vi "Flowmeter.vi"() -> ()   [LabVIEW 2018]
panel:
  in  "Doppler Flow Meter Graphs":u16(ring) items=["Ultrasound Speed", "Theta", "Frequency"]
  in  "Speed of Sound in Fluid (m/s)":dbl(knob) scale=0.0..1000.0
  out "XY Graph":cluster{"Y":dbl[], "Y":dbl[]}[](graph)
  in  "Switch 2":bool
  out "?":bool
  out "Velocity":dbl(knob) scale=0.0..5000.0
  in  "Ultrasonic Mode Switch":bool
  in  "?":bool
  in  "Thickness of pipe (mm)":dbl(slide) scale=0.0..200.0
  in  "Magnetic Field (T)":dbl(knob) scale=0.0..1000.0
  in  "Induced EMF (V)":dbl(knob) scale=0.0..10.0
  in  "Angle":dbl(knob) scale=90.0..30.0
  in  "Frequency 1 (KHz)":dbl(knob) scale=0.0..1000.0
  in  "Frequency 2 (KHz)":dbl(knob) scale=0.0..1000.0
  in  "milliseconds to wait":dbl
  in  "?":bool
  # "Variation wrt Difference\n      in Frequency"
  # "Variation wrt Angle"
  # "Electromagnetic"
  # "Ultrasonic"
  # "Doppler Flow Meter"
  # "Transit Time"
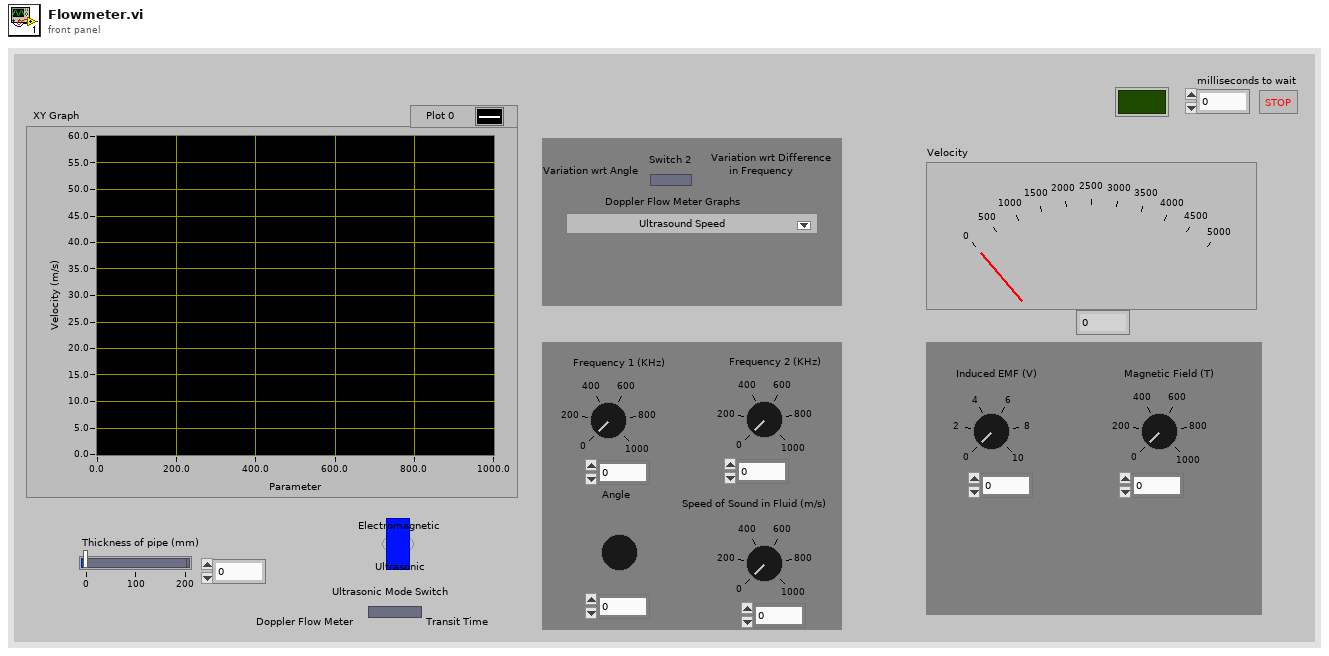
[diagram p1: front panel]
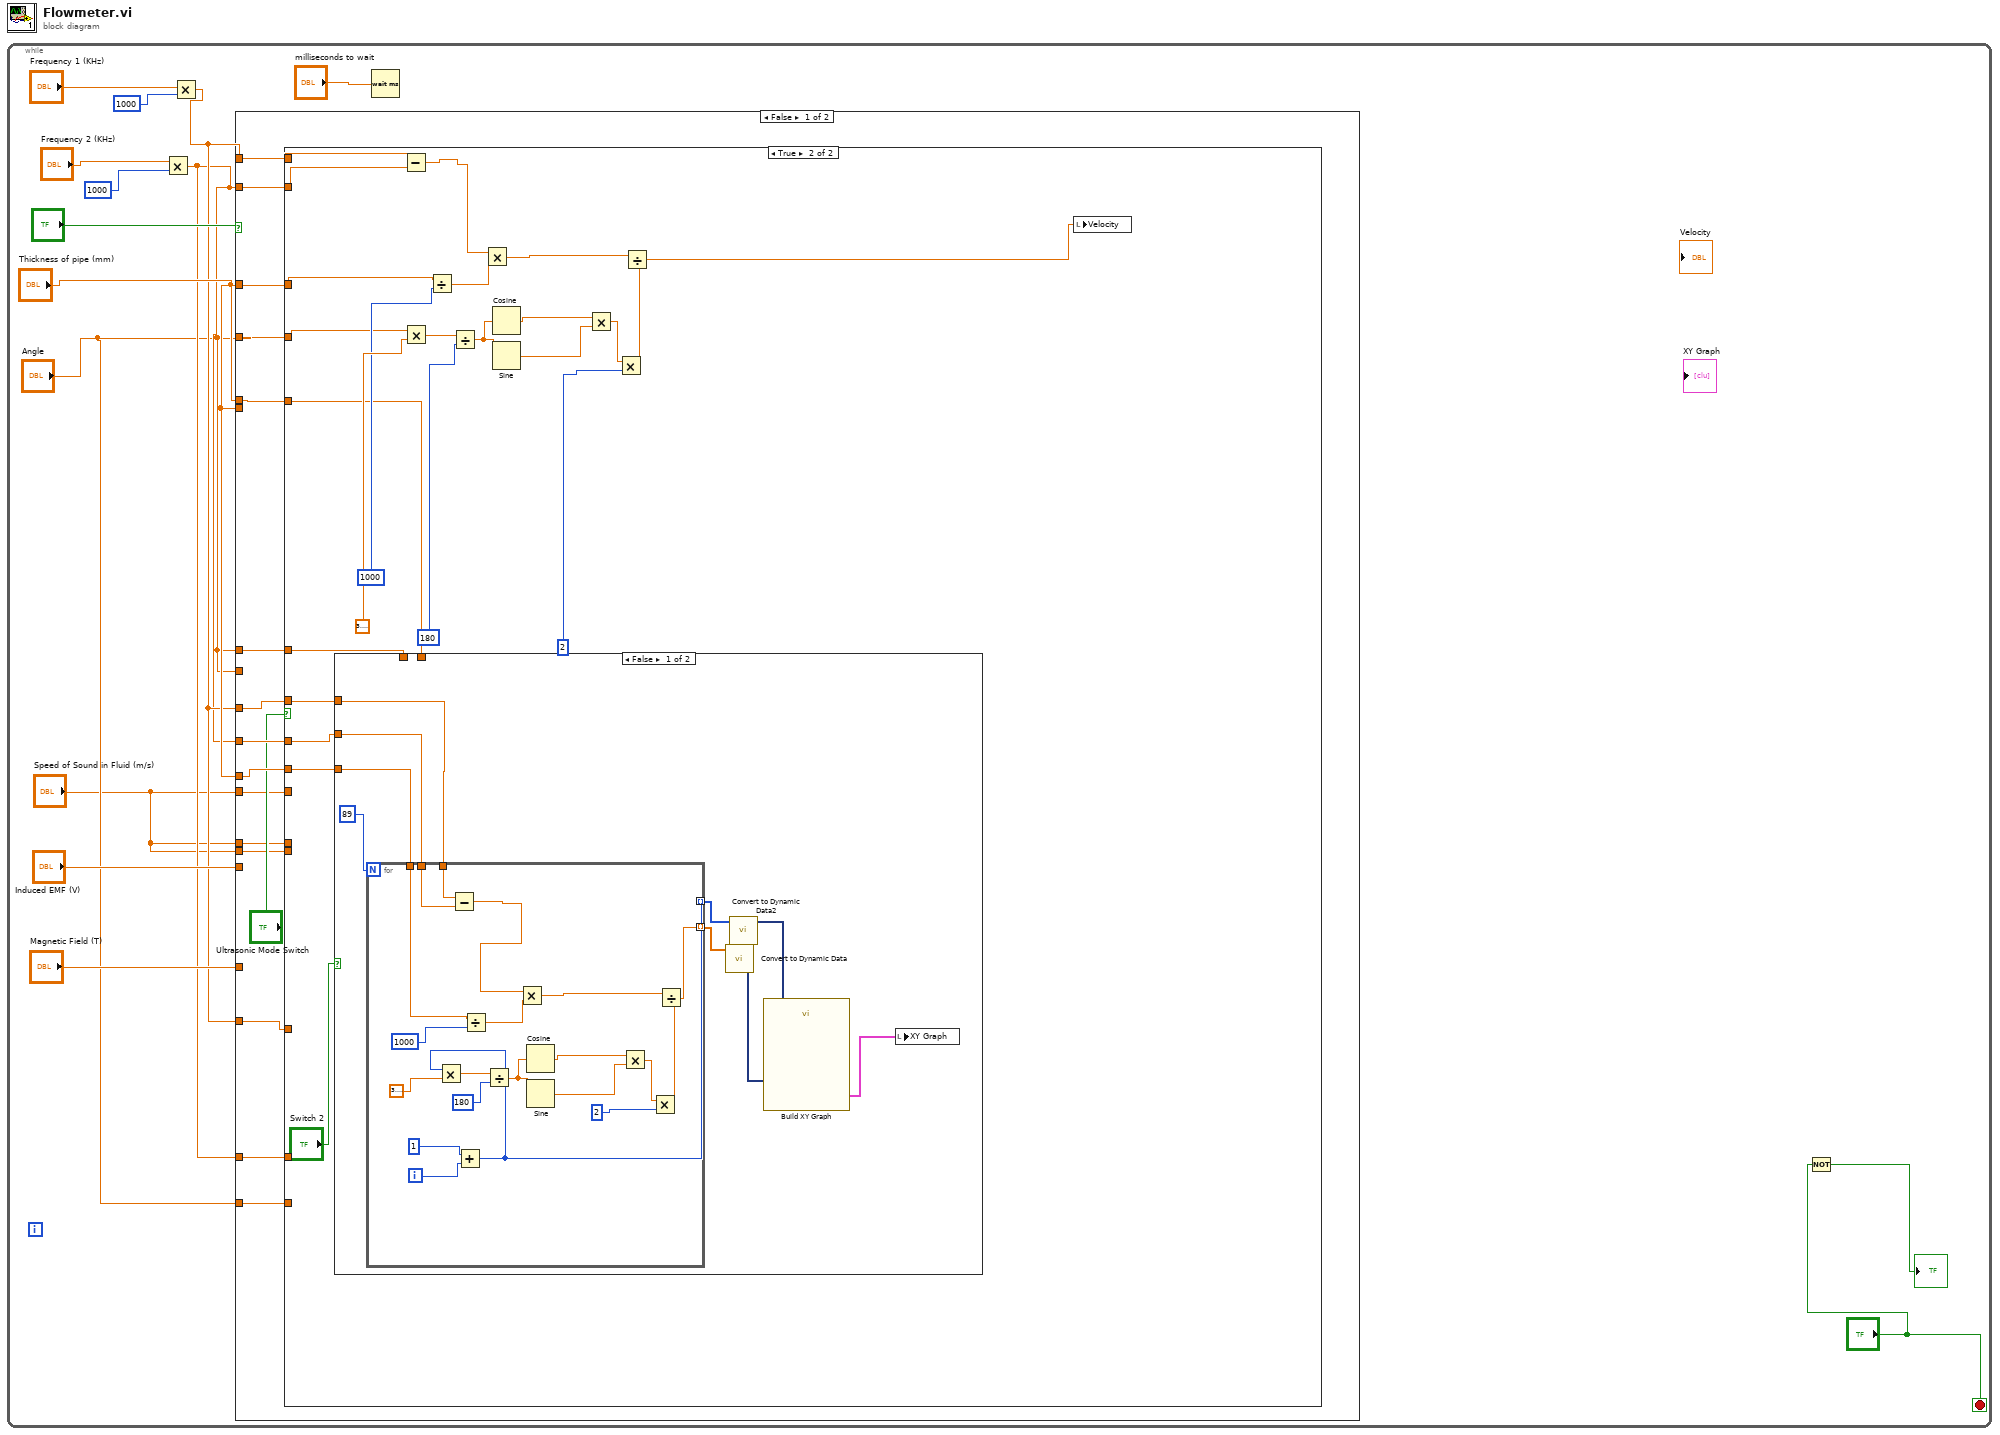
[diagram p0: block diagram]
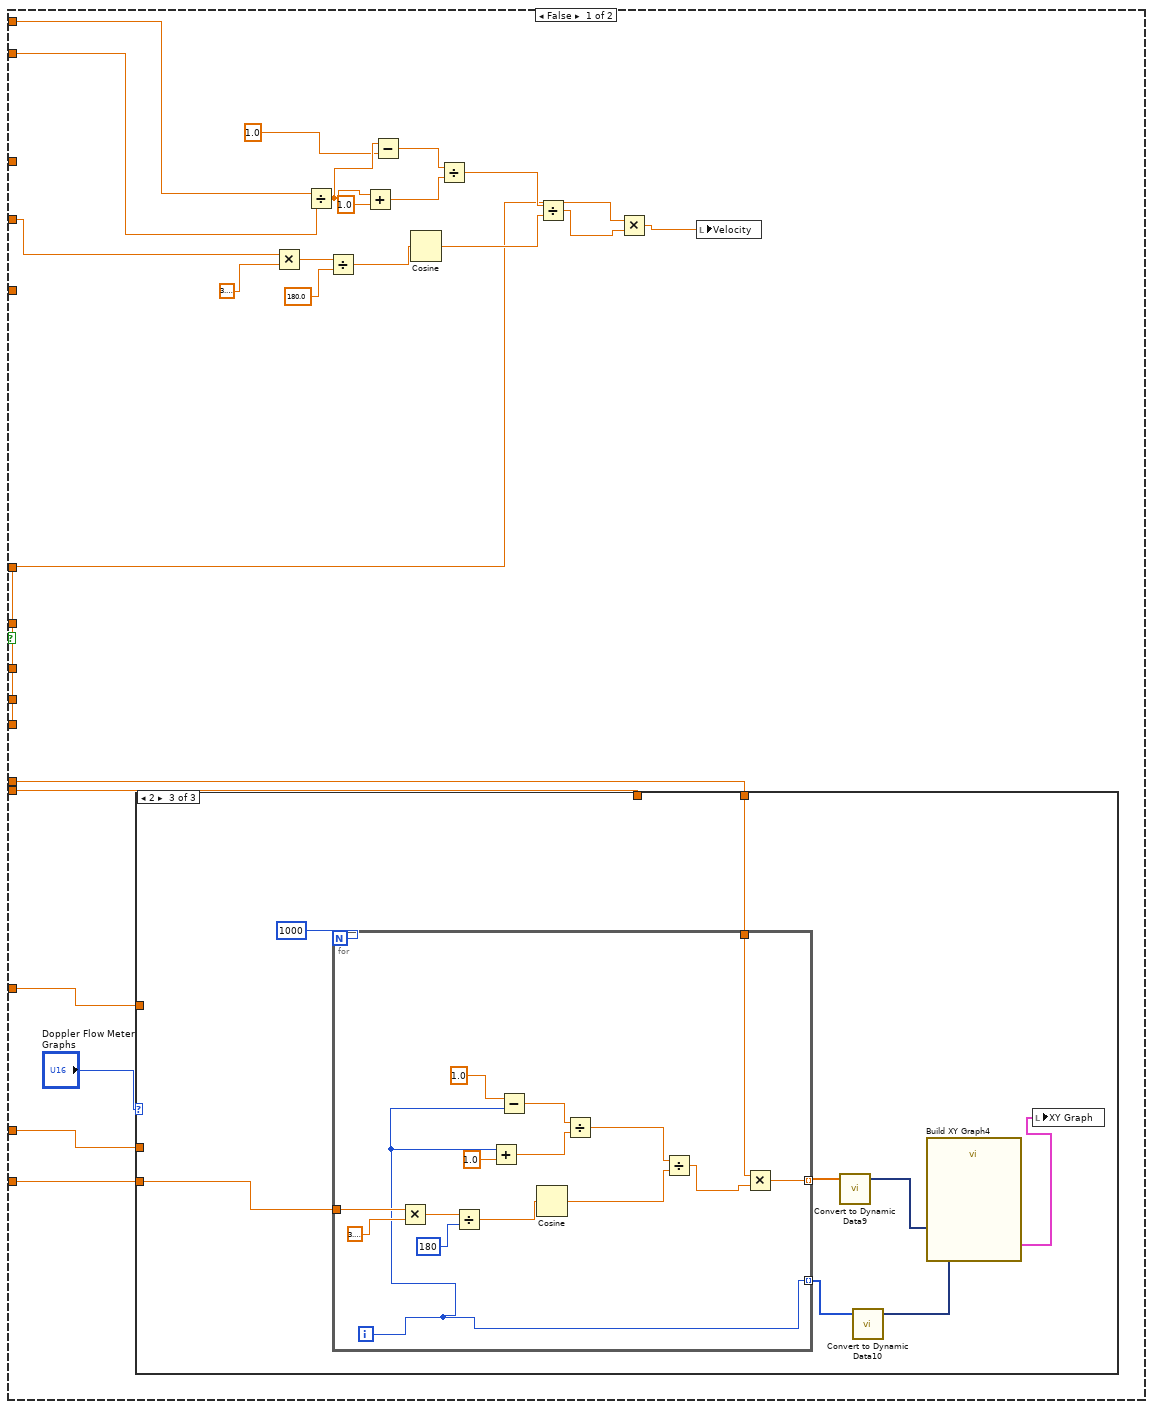
[diagram p2: hidden frame]
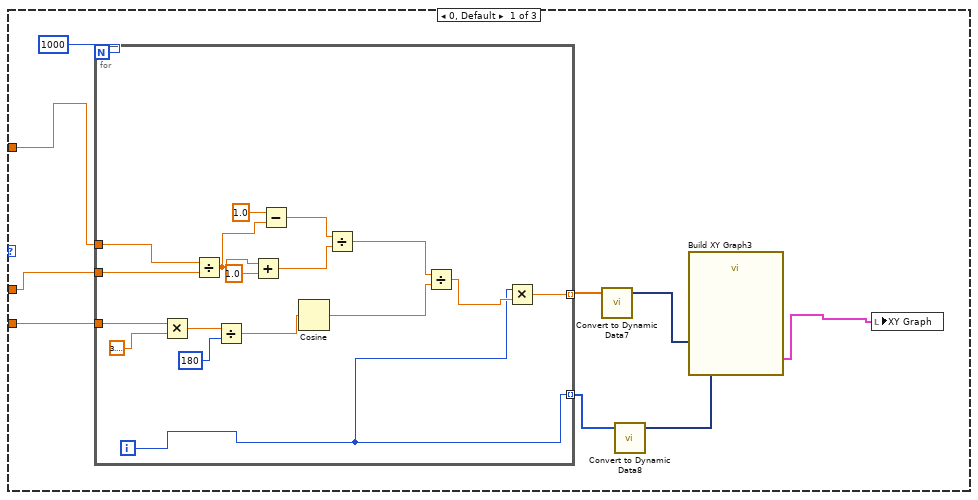
[diagram p3: hidden frame]
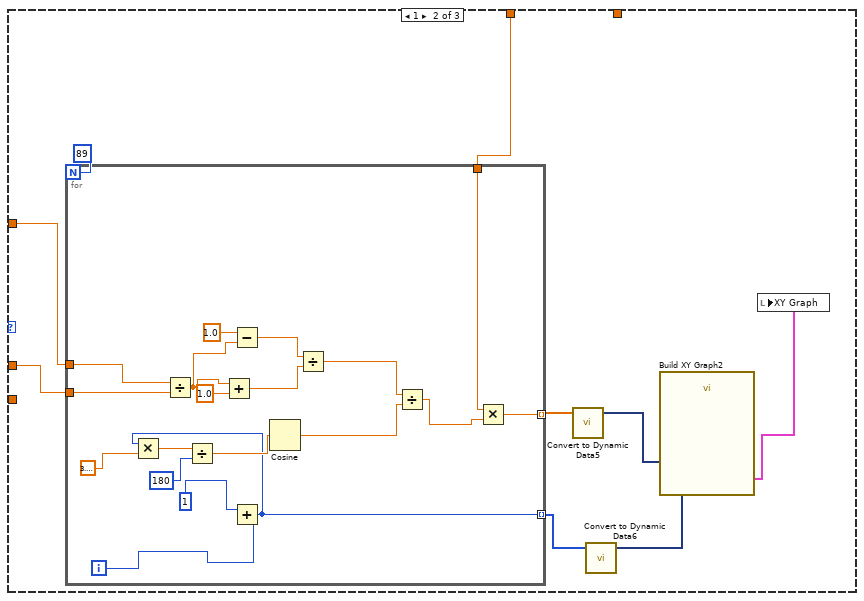
[diagram p4: hidden frame]
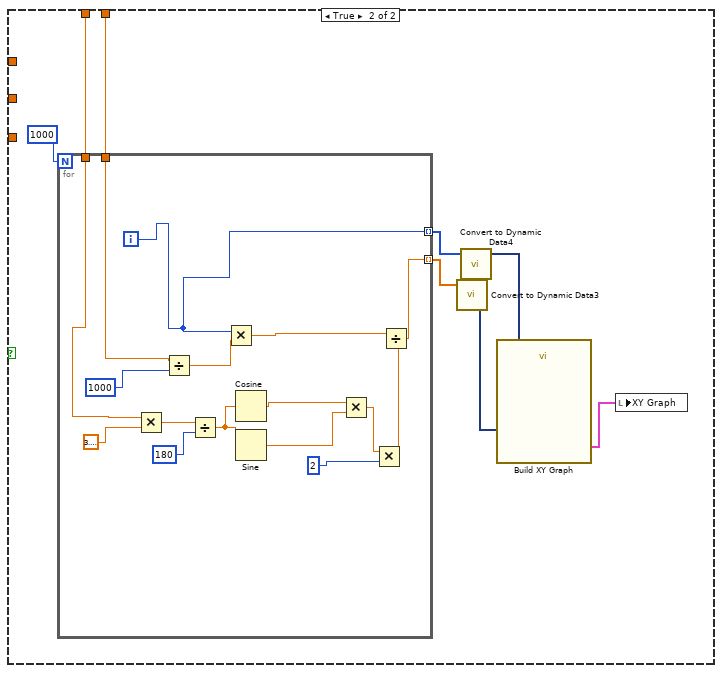
[diagram p5: hidden frame]
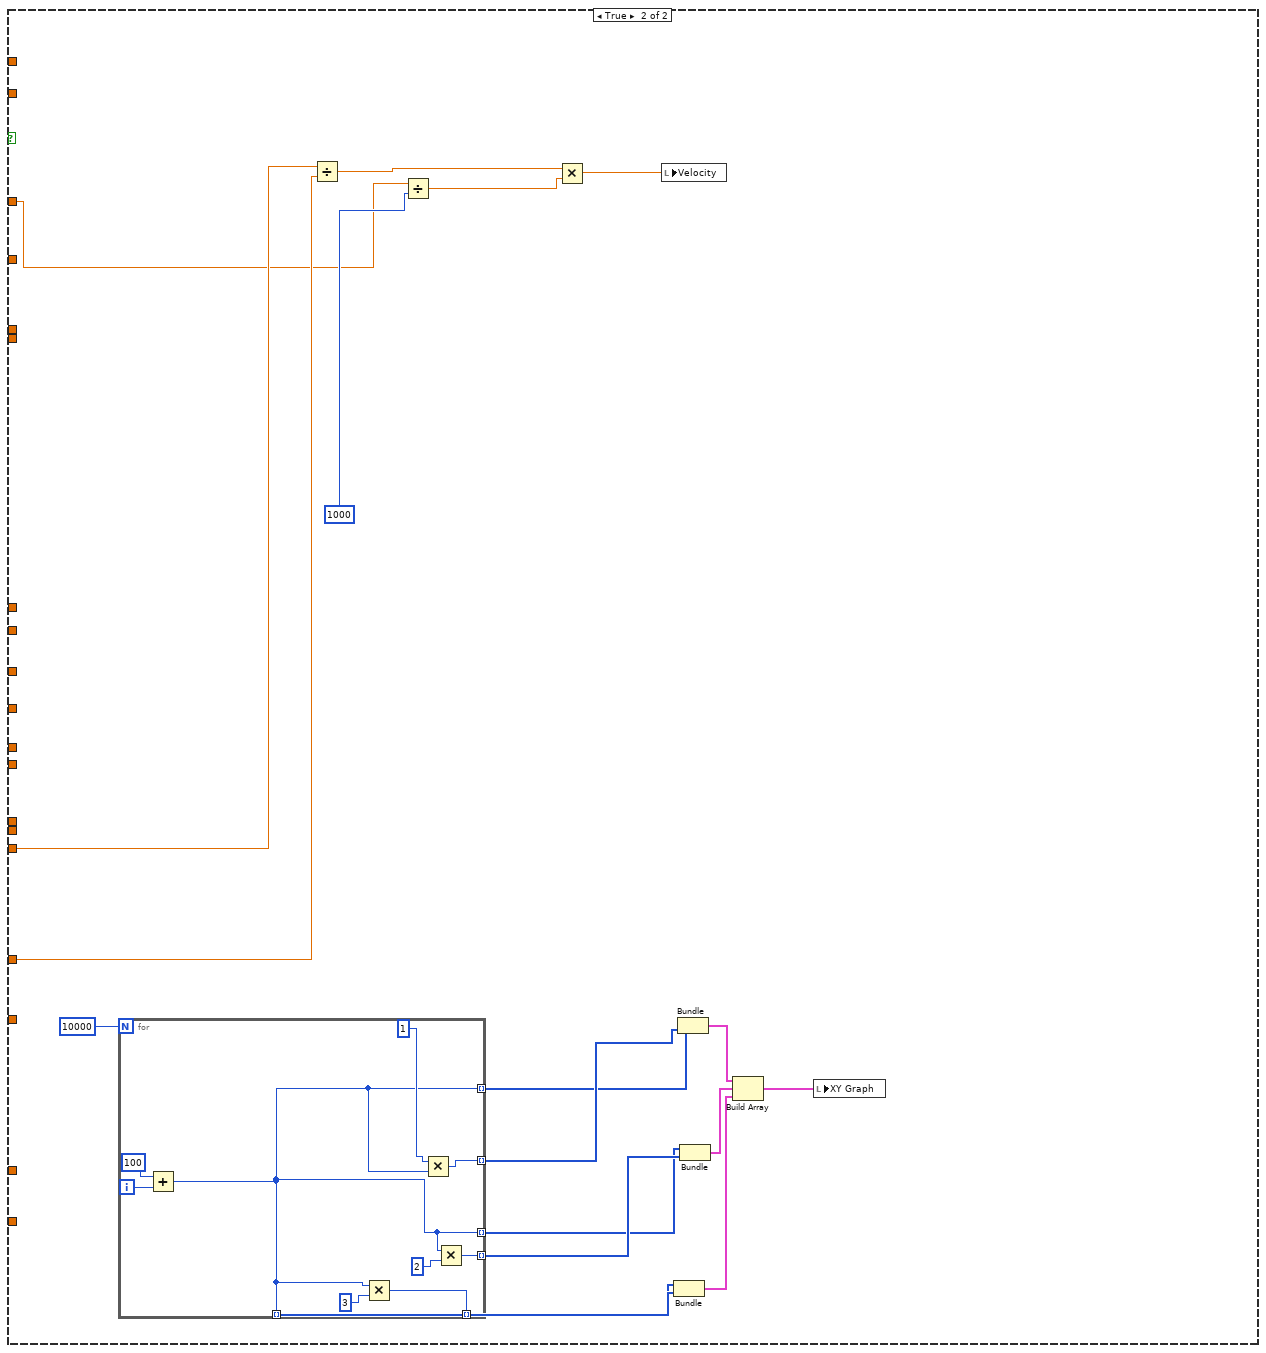
[diagram p6: hidden frame]
diagram:
  n1 = while {
    stop <- "?" stop-if-true
    n2 = Multiply(x="Frequency 2 (KHz)", y=1000) -> (x*y=w3:dbl)
    n3 = Multiply(x="Frequency 1 (KHz)", y=1000) -> (x*y=w4:dbl)
    n4 = case shown="False" "?" {
      tunnel: "Angle" -> [w28 _]
      tunnel: "Thickness of pipe (mm)" -> [w29 w221]
      tunnel: w3 -> [w30 _]
      tunnel: w4 -> [w31 _]
      tunnel: "Angle" -> [_ _]
      tunnel: "Thickness of pipe (mm)" -> [_ _]
      tunnel: "Thickness of pipe (mm)" -> [w25 _]
      tunnel: w4 -> [w27 _]
      tunnel: w3 -> [w26 _]
      tunnel: "Induced EMF (V)" -> [_ w223]
      tunnel: "Magnetic Field (T)" -> [_ w222]
      tunnel: "Thickness of pipe (mm)" -> [w23 _]
      tunnel: "Angle" -> [w22 _]
      tunnel: "Speed of Sound in Fluid (m/s)" -> [w21 _]
      tunnel: w4 -> [w20 _]
      tunnel: w3 -> [w19 _]
      tunnel: "Speed of Sound in Fluid (m/s)" -> [w18 _]
      tunnel: "Angle" -> [w17 _]
      tunnel: "Speed of Sound in Fluid (m/s)" -> [w16 _]
      frame False {
        n5 = case shown="True" "Ultrasonic Mode Switch" {
          tunnel: w31 -> [w42 w142]
          tunnel: w30 -> [w41 w141]
          tunnel: w29 -> [_ w140]
          tunnel: w28 -> [w40 w139]
          tunnel: w27 -> [_ w138]
          tunnel: w26 -> [_ w137]
          tunnel: w25 -> [_ w136]
          tunnel: w23 -> [_ w134]
          tunnel: w22 -> [_ w133]
          tunnel: w21 -> [w39 _]
          tunnel: w20 -> [w36 _]
          tunnel: w19 -> [w35 _]
          tunnel: w18 -> [w34 _]
          tunnel: w17 -> [w33 _]
          tunnel: w16 -> [w32 _]
          frame False {
            n6 = case shown="2" "Doppler Flow Meter Graphs" {
              tunnel: w36 -> [w58 w88 _]
              tunnel: w35 -> [w57 w87 _]
              tunnel: w34 -> [_ w86 _]
              tunnel: w33 -> [w56 _ w111]
              tunnel: w32 -> [_ _ w110]
              frame 0, Default {
                n7 = for {
                  N: 1000 -> [_]
                  tunnel: w58 -> [w73]
                  tunnel: w57 -> [w72]
                  tunnel: [w71] -> w59 mode=indexing
                  tunnel: [w64] -> w60 mode=indexing
                  tunnel: w56 -> [w65]
                  i -> [w64]
                  n8 = Multiply(x=w65, y=3.141592653589793) -> (x*y=w70:dbl)
                  n9 = Divide(x=w73, y=w72) -> (x/y=w66:dbl)
                  n10 = Divide(x=w70, y=180) -> (x/y=w67:dbl)
                  n11 = Add(x=w66, y=1.0) -> (x+y=w77:dbl)
                  n12 = Subtract(x=1.0, y=w66) -> (x-y=w78:dbl)
                  n13 = Cosine(x=w67) -> (cos(x)=w74:dbl)
                  n14 = Divide(x=w78, y=w77) -> (x/y=w76:dbl)
                  n15 = Divide(x=w76, y=w74) -> (x/y=w75:dbl)
                  n16 = Multiply(x=w64, y=w75) -> (x*y=w71:dbl)
                }
                n17 = call "Convert to Dynamic Data7"("Array"=w59) -> ("Dynamic Data Type"=w61:dynamicdata)  [unwired: 3 in]
                n18 = call "Convert to Dynamic Data8"("Array"=w60) -> ("Dynamic Data Type"=w62:dynamicdata)  [unwired: 3 in]
                n19 = call "Build XY Graph3"("Y Input"=w61, "X Input"=w62) -> ("XY Graph"=w55:cluster{"X":dbl[], "Y":dbl[]}[])  [unwired: 8 in, 1 out]
                n20 = local write "XY Graph"(w55) -> ()
              }
              frame 1 {
                n21 = for {
                  N: 89 -> [_]
                  tunnel: w88 -> [w101]
                  tunnel: w87 -> [w100]
                  tunnel: [w99] -> w82 mode=indexing
                  tunnel: [w90] -> w83 mode=indexing
                  tunnel: w86 -> [w91]
                  i -> [w98]
                  n22 = Divide(x=w101, y=w100) -> (x/y=w92:dbl)
                  n23 = Add(x=w92, y=1.0) -> (x+y=w105:dbl)
                  n24 = Subtract(x=1.0, y=w92) -> (x-y=w106:dbl)
                  n25 = Add(x=1, y=w98) -> (x+y=w90:i32)
                  n26 = Multiply(x=w90, y=3.141592653589793) -> (x*y=w96:dbl)
                  n27 = Divide(x=w96, y=180) -> (x/y=w93:dbl)
                  n28 = Cosine(x=w93) -> (cos(x)=w102:dbl)
                  n29 = Divide(x=w106, y=w105) -> (x/y=w104:dbl)
                  n30 = Divide(x=w104, y=w102) -> (x/y=w103:dbl)
                  n31 = Multiply(x=w91, y=w103) -> (x*y=w99:dbl)
                }
                n32 = call "Convert to Dynamic Data5"("Array"=w82) -> ("Dynamic Data Type"=w84:dynamicdata)  [unwired: 3 in]
                n33 = call "Convert to Dynamic Data6"("Array"=w83) -> ("Dynamic Data Type"=w85:dynamicdata)  [unwired: 3 in]
                n34 = call "Build XY Graph2"("Y Input"=w84, "X Input"=w85) -> ("XY Graph"=w81:cluster{"X":dbl[], "Y":dbl[]}[])  [unwired: 8 in, 1 out]
                n35 = local write "XY Graph"(w81) -> ()
              }
              frame 2 {
                n36 = for {
                  N: 1000 -> [_]
                  tunnel: [w124] -> w112 mode=indexing
                  tunnel: [w117] -> w113 mode=indexing
                  tunnel: w111 -> [w119]
                  tunnel: w110 -> [w118]
                  i -> [w117]
                  n37 = Multiply(x=w119, y=3.141592653589793) -> (x*y=w123:dbl)
                  n38 = Divide(x=w123, y=180) -> (x/y=w120:dbl)
                  n39 = Add(x=w117, y=1.0) -> (x+y=w128:dbl)
                  n40 = Subtract(x=1.0, y=w117) -> (x-y=w129:dbl)
                  n41 = Cosine(x=w120) -> (cos(x)=w125:dbl)
                  n42 = Divide(x=w129, y=w128) -> (x/y=w127:dbl)
                  n43 = Divide(x=w127, y=w125) -> (x/y=w126:dbl)
                  n44 = Multiply(x=w118, y=w126) -> (x*y=w124:dbl)
                }
                n45 = call "Convert to Dynamic Data9"("Array"=w112) -> ("Dynamic Data Type"=w114:dynamicdata)  [unwired: 3 in]
                n46 = call "Convert to Dynamic Data10"("Array"=w113) -> ("Dynamic Data Type"=w115:dynamicdata)  [unwired: 3 in]
                n47 = call "Build XY Graph4"("Y Input"=w114, "X Input"=w115) -> ("XY Graph"=w109:cluster{"X":dbl[], "Y":dbl[]}[])  [unwired: 8 in, 1 out]
                n48 = local write "XY Graph"(w109) -> ()
              }
            }
            n49 = Multiply(x=w40, y=3.141592653589793) -> (x*y=w48:dbl)
            n50 = Divide(x=w42, y=w41) -> (x/y=w44:dbl)
            n51 = Divide(x=w48, y=180.0) -> (x/y=w47:dbl)
            n52 = Add(x=w44, y=1.0) -> (x+y=w52:dbl)
            n53 = Subtract(x=w44, y=1.0 ("x")) -> (x-y=w53:dbl)
            n54 = Cosine(x=w47) -> (cos(x)=w49:dbl)
            n55 = Divide(x=w53, y=w52) -> (x/y=w51:dbl)
            n56 = Divide(x=w51, y=w49) -> (x/y=w50:dbl)
            n57 = Multiply(x=w39, y=w50) -> (x*y=w38:dbl)
            n58 = local write "Velocity"(w38) -> ()
          }
          frame True {
            n59 = case shown="False" "Switch 2" {
              tunnel: w133 -> [_ w187]
              tunnel: w134 -> [_ w186]
              tunnel: w136 -> [w159 _]
              tunnel: w138 -> [w158 _]
              tunnel: w137 -> [w157 _]
              frame False {
                n60 = for {
                  N: 89 -> [_]
                  tunnel: w159 -> [w172]
                  tunnel: w158 -> [w170]
                  tunnel: [w166] -> w160 mode=indexing
                  tunnel: [w171] -> w161 mode=indexing
                  tunnel: w157 -> [w169]
                  i -> [w168]
                  n61 = Subtract(x=w170, y=w169) -> (x-y=w165:dbl)
                  n62 = Add(x=1, y=w168) -> (x+y=w166:i32)
                  n63 = Multiply(x=w166, y=3.141592653589793) -> (x*y=w177:dbl)
                  n64 = Divide(x=w172, y=1000) -> (x/y=w184:dbl)
                  n65 = Divide(x=w177, y=180) -> (x/y=w178:dbl)
                  n66 = Multiply(x=w165, y=w184) -> (x*y=w182:dbl)
                  n67 = Cosine(x=w178) -> (cos(x)=w179:dbl)
                  n68 = Sine(x=w178) -> (sin(x)=w180:dbl)
                  n69 = Multiply(x=w179, y=w180) -> (x*y=w181:dbl)
                  n70 = Multiply(x=w181, y=2) -> (x*y=w183:dbl)
                  n71 = Divide(x=w182, y=w183) -> (x/y=w171:dbl)
                }
                n72 = call "Convert to Dynamic Data"("Array"=w161) -> ("Dynamic Data Type"=w163:dynamicdata)  [unwired: 3 in]
                n73 = call "Convert to Dynamic Data2"("Array"=w160) -> ("Dynamic Data Type"=w162:dynamicdata)  [unwired: 3 in]
                n74 = call "Build XY Graph"("Y Input"=w163, "X Input"=w162) -> ("XY Graph"=w156:cluster{"X":dbl[], "Y":dbl[]}[])  [unwired: 8 in, 1 out]
                n75 = local write "XY Graph"(w156) -> ()
              }
              frame True {
                n76 = for {
                  N: 1000 -> [_]
                  tunnel: w186 -> [w196]
                  tunnel: w187 -> [w195]
                  tunnel: [w193] -> w188 mode=indexing
                  tunnel: [w194] -> w189 mode=indexing
                  i -> [w193]
                  n77 = Multiply(x=w195, y=3.141592653589793) -> (x*y=w201:dbl)
                  n78 = Divide(x=w196, y=1000) -> (x/y=w208:dbl)
                  n79 = Divide(x=w201, y=180) -> (x/y=w202:dbl)
                  n80 = Multiply(x=w193, y=w208) -> (x*y=w206:dbl)
                  n81 = Cosine(x=w202) -> (cos(x)=w203:dbl)
                  n82 = Sine(x=w202) -> (sin(x)=w204:dbl)
                  n83 = Multiply(x=w203, y=w204) -> (x*y=w205:dbl)
                  n84 = Multiply(x=w205, y=2) -> (x*y=w207:dbl)
                  n85 = Divide(x=w206, y=w207) -> (x/y=w194:dbl)
                }
                n86 = call "Convert to Dynamic Data3"("Array"=w189) -> ("Dynamic Data Type"=w191:dynamicdata)  [unwired: 3 in]
                n87 = call "Convert to Dynamic Data4"("Array"=w188) -> ("Dynamic Data Type"=w190:dynamicdata)  [unwired: 3 in]
                n88 = call "Build XY Graph"("Y Input"=w191, "X Input"=w190) -> ("XY Graph"=w185:cluster{"X":dbl[], "Y":dbl[]}[])  [unwired: 8 in, 1 out]
                n89 = local write "XY Graph"(w185) -> ()
              }
            }
            n90 = Subtract(x=w142, y=w141) -> (x-y=w143:dbl)
            n91 = Multiply(x=w139, y=3.141592653589793) -> (x*y=w153:dbl)
            n92 = Divide(x=w140, y=1000) -> (x/y=w144:dbl)
            n93 = Divide(x=w153, y=180) -> (x/y=w151:dbl)
            n94 = Multiply(x=w143, y=w144) -> (x*y=w147:dbl)
            n95 = Cosine(x=w151) -> (cos(x)=w150:dbl)
            n96 = Sine(x=w151) -> (sin(x)=w149:dbl)
            n97 = Multiply(x=w150, y=w149) -> (x*y=w148:dbl)
            n98 = Multiply(x=w148, y=2) -> (x*y=w146:dbl)
            n99 = Divide(x=w147, y=w146) -> (x/y=w132:dbl)
            n100 = local write "Velocity"(w132) -> ()
          }
        }
      }
      frame True {
        n101 = for {
          N: 10000 -> [_]
          tunnel: [w229] -> w219 mode=indexing
          tunnel: [w233] -> w220 mode=indexing
          tunnel: [w229] -> w215 mode=indexing
          tunnel: [w229] -> w217 mode=indexing
          tunnel: [w230] -> w216 mode=indexing
          tunnel: [w227] -> w218 mode=indexing
          i -> [w235]
          n102 = Add(x=100, y=w235) -> (x+y=w229:i32)
          n103 = Multiply(x=w229, y=3) -> (x*y=w227:i32)
          n104 = Multiply(x=1, y=w229) -> (x*y=w233:i32)
          n105 = Multiply(x=w229, y=2) -> (x*y=w230:i32)
        }
        n106 = Divide(x=w223, y=w222) -> (x/y=w226:dbl)
        n107 = Divide(x=w221, y=1000) -> (x/y=w224:dbl)
        n108 = Multiply(x=w226, y=w224) -> (x*y=w210:dbl)
        n109 = local write "Velocity"(w210) -> ()
        n110 = Bundle(w217, w218) -> (w214:cluster{i32[], i32[]})  [unwired: 1 in]
        n111 = Bundle(w219, w220) -> (w212:cluster{i32[], i32[]})  [unwired: 1 in]
        n112 = Bundle(w215, w216) -> (w213:cluster{i32[], i32[]})  [unwired: 1 in]
        n113 = Build Array(w212, w213, w214) -> (w209:cluster{i32[], i32[]}[])
        n114 = local write "XY Graph"(w209) -> ()
      }
    }
    n115 = Wait (ms)(milliseconds to wait="milliseconds to wait") -> ()  [unwired: 1 out]
    n116 = Not(x="?") -> (.not. x?=→"?":bool)
  }
